vi "RampToZero.vi"(6 "sampling info":cluster{"Fs":dbl, "#s":dbl}={"Fs"=1000.0, "#s"=1000.0} {"Fs" format="%.2p"}, 8 "error in (no error)":errorcluster, 11 "starting value":dbl=1.0 format="%.2p") -> (0 "error out":errorcluster, 2 "Waveform Graph":waveform(dbl)(graph))   [LabVIEW 2016, in "Generator.lvclass"]
uses:
  Generator.lvclass
  <vilib>/Analysis/NI_AALBase.lvlib
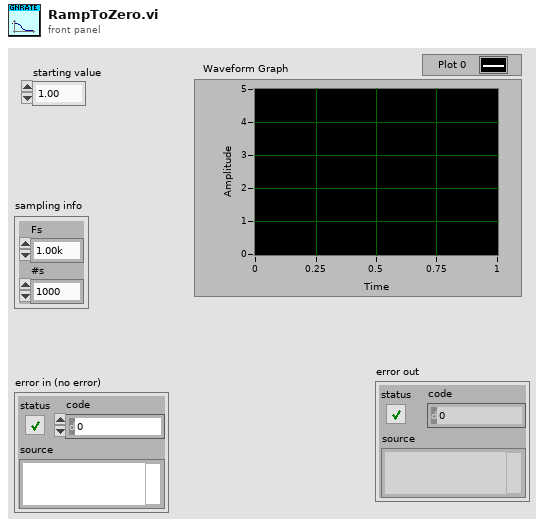
[diagram p1: front panel]
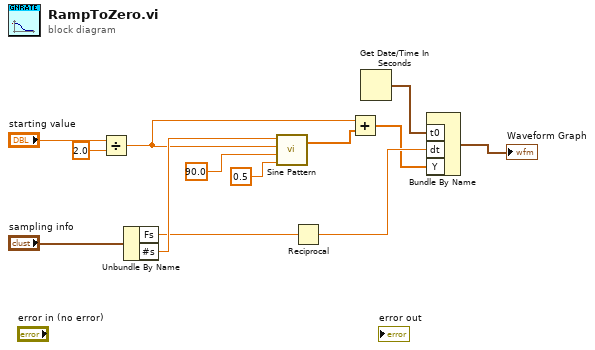
[diagram p0: block diagram]
diagram:
  n1 = Divide(x="starting value", y=2.0) -> (x/y=w6:dbl)
  n2 = Unbundle By Name("sampling info") -> ("Fs"=w4:dbl, "#s"=w9:dbl)
  n3 = call <vilib>:"Sine Pattern.vi"("cycles"=0.5, "phase(degrees)"=90.0 ("y"), "amplitude"=w6, "samples"=w9) -> ("Sinusoidal Pattern"=w3:dbl[])  [unwired: 1 out]
  n4 = Reciprocal(x=w4) -> (1/x=w8:dbl)
  n5 = Add(x=w6, y=w3) -> (x+y=w5:dbl[])
  n6 = Get Date/Time In Seconds() -> (seconds since 1Jan1904=w1:timestamp)
  n7 = Bundle By Name("t0"=w1, "dt"=w8, "Y"=w5) -> (→"Waveform Graph":waveform(dbl))  [unwired: 1 in]
